vi "I2C SDA In.vi"(9 "SDA_IN":bool, 10 "Sample":bool, 11 "Reset":bool) -> (3 "Data Out":u8)   [LabVIEW 2016]
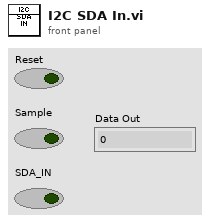
[diagram p1: front panel]
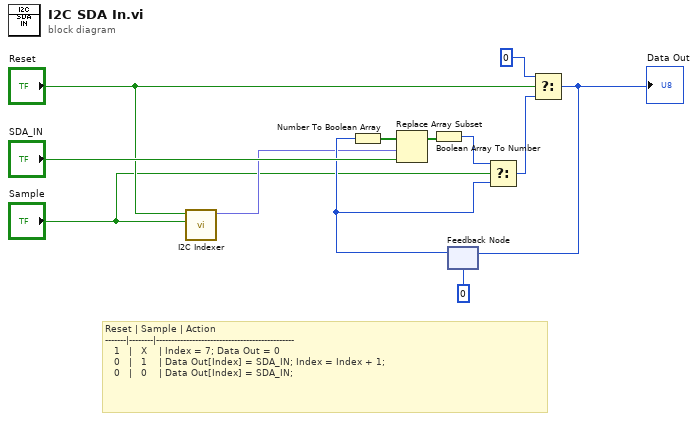
[diagram p0: block diagram]
diagram:
  # "Reset | Sample | Action\n-------|--------|----------------------------------------------\n   1   |   X    | Index = 7; Data Out = 0\n   0   |   1    | Data Out[Index] = SDA_IN; Index = Index + 1;\n   0   |   0    | Data Out[Index] = SDA_IN;"
  n1 = call "I2C Indexer.vi"("Decrement?"="Sample", "Load?"="Reset") -> ("Numeric"=w3:fxp<+,3,3>)  [unwired: 9 in]
  n2 = feedback #1(u8 0 ("Data Out")) -> (w7:u8)
  n3 = Number To Boolean Array(number=w7) -> (Boolean array=w11:bool[])
  n4 = Replace Array Subset(array=w11, new element="SDA_IN", index=w3) -> (w9:bool[])
  n5 = Boolean Array To Number(Boolean array=w9) -> (number=w8:u8)
  n6 = Select(t=w8, s="Sample", f=w7) -> (s? t:f=w5:u8)
  n7 = Select(t=u8 0 ("Data Out"), s="Reset", f=w5) -> (s? t:f=w4:u8)
  "Data Out" <- w4
  n8 = feedback-in #1(w4) -> ()
